vi "Initialize.vi"(7 "Option String":string="Simulate=1,RangeCheck=1,QueryInstrStatus=1,Cache=0", 8 "error in (no error)":errorcluster, 9 "btnReset":bool caption="Reset (F)", 10 "btnIdQuery":bool caption="Id Query (F)", 11 "ChromaAcLoad in":refnum<class "ChromaAcLoad.lvclass">) -> (0 "error out":errorcluster, 3 "ChromaAcLoad out":refnum<class "ChromaAcLoad.lvclass">)   [LabVIEW 2018, in "AcPwrPlugins.lvlib" / "ChromaAcLoad.lvclass"]
doc: "This VI estabilishes communication ot the instrument and optionally sets the initial state of the following session attributes:\n\n C63800_ATTR_RANGE_CHECK \n C63800_ATTR_QUERY_INSTR_STATUS \n C63800_ATTR_CACHE \n C63800_ATTR_SIMULATE \n C63800_ATTR_RECORD_COERCIONS \n\n- Opens a session to the specified device using the interface and address you specify for the Resource Name parameter.\n\n- If the ID Query parameter is set to VI_TRUE, this function queries the instrument ID and checks that it is valid for this instrument driver.\n\n- If the Reset parameter is set to VI_TRUE, this function resets the instrument to a known state.\n\n- Sends initialization commands to set the instrument to the state necessary for the operation of the instrument driver.\n\n- Returns a ViSession handle that you use to identify the instrument in all subsequent instrument driver function calls.\n\nNote: This function creates a new session each time you invoke it. Although you can open more than one IVI session for the same resource, it is best not to do so. You can use the same session in multiple program threads. You can use the C63800_LockSession and C63800_UnlockSession functions to protect sections of code that require exclusive access to the resource."
uses:
  ChromaAcLoad.lvclass
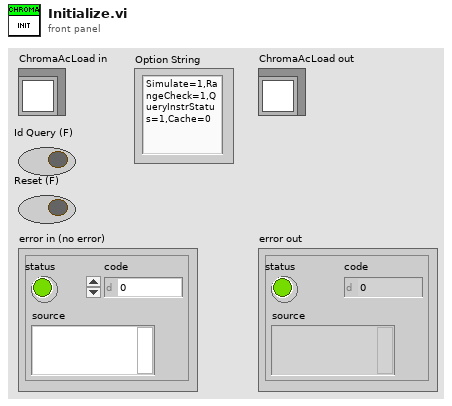
[diagram p1: front panel]
types:
  T1 = cluster{"f":bool, "Instrument Handle out":refnum<k15>}[]
  T2 = typedef "AcPwrPlugins.lvlib/ChromaAcLoad.lvclass/DeviceProperties.ctl" = cluster{"Frequency (Hz)":dbl, "Phases":cluster{"Handle":string, "Name":string, "Phase Select":i32, "option string ":string, "id query (Yes)":bool, "reset device (Yes)":bool, "LC":cluster{"C (uF)":i32, "L (uH)":i32, "RS (Ohm)":dbl, "RL (Ohm)":dbl}, "Load Current (A/Arms)":dbl, "Load Voltage (V/Vrms)":dbl, "Load Power (W)":dbl, "Load Resistance (Ohms)":dbl, "Load Current Peak (A)":dbl, "Load Current Limit (A/Arms)":dbl, "Slew Rate":cluster{"Rise Slew Rate (Units/S)":i32, "Fall Slew Rate (Units/S)":i32}, "Load Short Circuited":bool, "Line Synchronization":bool, "Priority":enum16{"CF Only", "PF Only", "Both (CF)", "Both (PF)"}, "Crest Factor":dbl, "Power Factor":dbl, "Connected":bool, "Voltage Range (V)":dbl[], "Timing":cluster{"TimingOn":enum16{""}, "Hours":u32, "Minutes":u32, "Seconds":dbl, "CutoffVoltage":dbl}}[], "Configuration Mode":enum16{"Constant Voltage (DC)", "Constant Power (DC)", "Constant Power (AC)", "Constant Current (DC)", "Constant Current (AC)", "Constant Resistance (DC)", "Constant Resistance (AC)", "Rectified Mode (DC)", "Inrush (AC)", "RLC CP (AC)", "RLC (AC)"}}[]
  T3 = cluster{"Handle":string, "Name":string, "Phase Select":i32, "option string ":string, "id query (Yes)":bool, "reset device (Yes)":bool, "LC":cluster{"C (uF)":i32, "L (uH)":i32, "RS (Ohm)":dbl, "RL (Ohm)":dbl}, "Load Current (A/Arms)":dbl, "Load Voltage (V/Vrms)":dbl, "Load Power (W)":dbl, "Load Resistance (Ohms)":dbl, "Load Current Peak (A)":dbl, "Load Current Limit (A/Arms)":dbl, "Slew Rate":cluster{"Rise Slew Rate (Units/S)":i32, "Fall Slew Rate (Units/S)":i32}, "Load Short Circuited":bool, "Line Synchronization":bool, "Priority":enum16{"CF Only", "PF Only", "Both (CF)", "Both (PF)"}, "Crest Factor":dbl, "Power Factor":dbl, "Connected":bool, "Voltage Range (V)":dbl[], "Timing":cluster{"TimingOn":enum16{""}, "Hours":u32, "Minutes":u32, "Seconds":dbl, "CutoffVoltage":dbl}}[]
  T4 = cluster{"f":bool, "Instrument Handle out":refnum<k15>}
  T5 = cluster{"Handle":string, "Name":string, "Phase Select":i32, "option string ":string, "id query (Yes)":bool, "reset device (Yes)":bool, "LC":cluster{"C (uF)":i32, "L (uH)":i32, "RS (Ohm)":dbl, "RL (Ohm)":dbl}, "Load Current (A/Arms)":dbl, "Load Voltage (V/Vrms)":dbl, "Load Power (W)":dbl, "Load Resistance (Ohms)":dbl, "Load Current Peak (A)":dbl, "Load Current Limit (A/Arms)":dbl, "Slew Rate":cluster{"Rise Slew Rate (Units/S)":i32, "Fall Slew Rate (Units/S)":i32}, "Load Short Circuited":bool, "Line Synchronization":bool, "Priority":enum16{"CF Only", "PF Only", "Both (CF)", "Both (PF)"}, "Crest Factor":dbl, "Power Factor":dbl, "Connected":bool, "Voltage Range (V)":dbl[], "Timing":cluster{"TimingOn":enum16{""}, "Hours":u32, "Minutes":u32, "Seconds":dbl, "CutoffVoltage":dbl}}
  T6 = cluster{"Frequency (Hz)":dbl, "Phases":cluster{"Handle":string, "Name":string, "Phase Select":i32, "option string ":string, "id query (Yes)":bool, "reset device (Yes)":bool, "LC":cluster{"C (uF)":i32, "L (uH)":i32, "RS (Ohm)":dbl, "RL (Ohm)":dbl}, "Load Current (A/Arms)":dbl, "Load Voltage (V/Vrms)":dbl, "Load Power (W)":dbl, "Load Resistance (Ohms)":dbl, "Load Current Peak (A)":dbl, "Load Current Limit (A/Arms)":dbl, "Slew Rate":cluster{"Rise Slew Rate (Units/S)":i32, "Fall Slew Rate (Units/S)":i32}, "Load Short Circuited":bool, "Line Synchronization":bool, "Priority":enum16{"CF Only", "PF Only", "Both (CF)", "Both (PF)"}, "Crest Factor":dbl, "Power Factor":dbl, "Connected":bool, "Voltage Range (V)":dbl[], "Timing":cluster{"TimingOn":enum16{""}, "Hours":u32, "Minutes":u32, "Seconds":dbl, "CutoffVoltage":dbl}}[], "Configuration Mode":enum16{"Constant Voltage (DC)", "Constant Power (DC)", "Constant Power (AC)", "Constant Current (DC)", "Constant Current (AC)", "Constant Resistance (DC)", "Constant Resistance (AC)", "Rectified Mode (DC)", "Inrush (AC)", "RLC CP (AC)", "RLC (AC)"}}
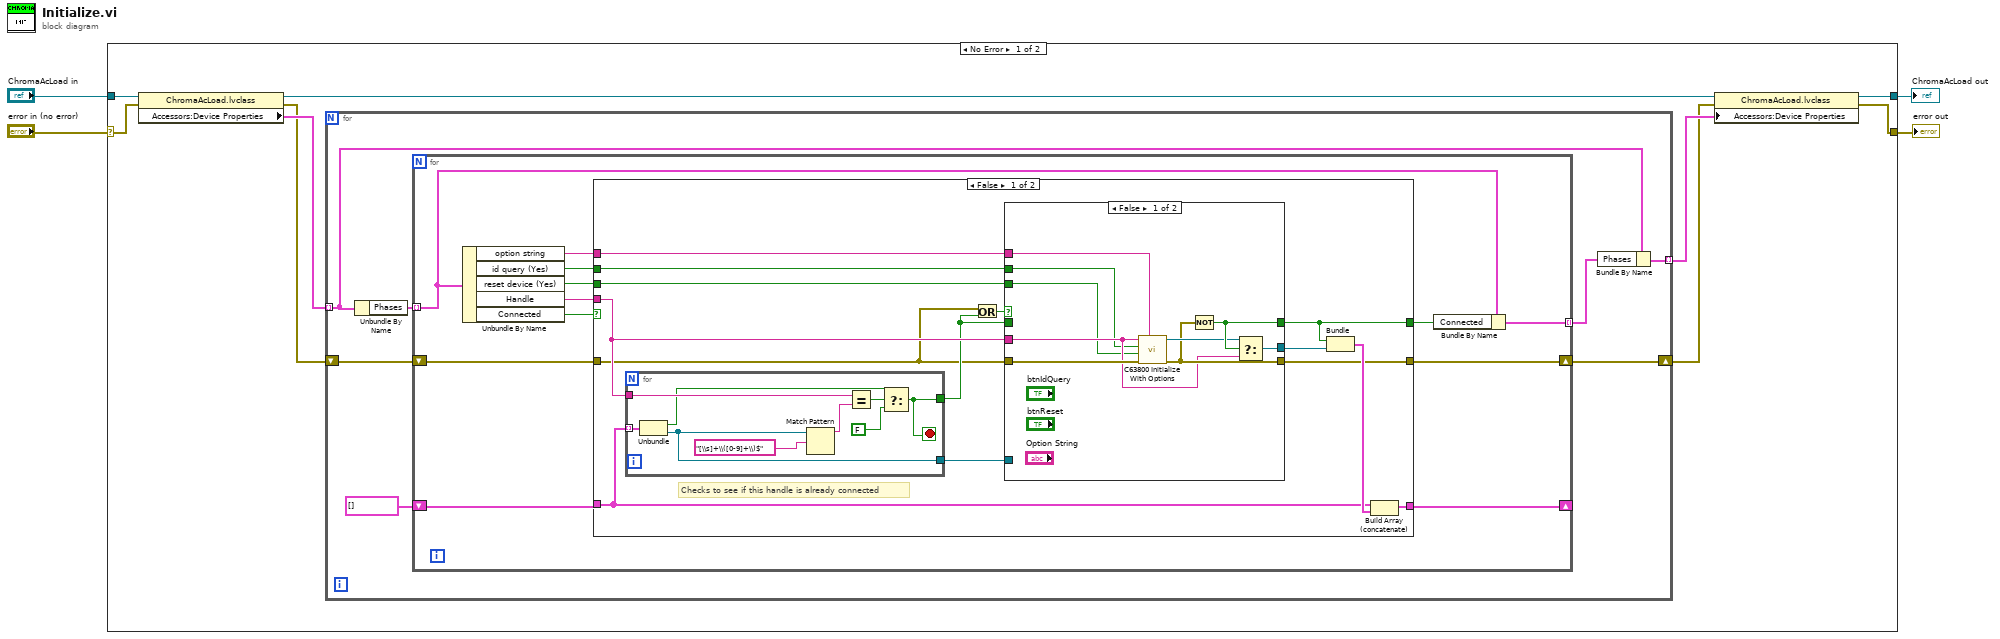
[diagram p0: block diagram]
diagram:
  n1 = case shown="No Error" "error in (no error)" {
    selector: "error in (no error)" -> [w12 w72]
    tunnel: "ChromaAcLoad in" -> [w13 w71]
    tunnel: [w10 w71] -> w2
    tunnel: [w5 w72] -> w1
    frame No Error {
      n2 = property class="ChromaAcLoad.lvclass"(reference=w13, error in=w12) -> (reference out=w11:refnum<class "ChromaAcLoad.lvclass">, error out=w7:errorcluster, "Accessors:Device Properties"=w9:T2)
      n3 = for {
        tunnel: w9 -> [w20] mode=indexing
        tunnel: [w19] -> w8 mode=indexing
        shift-right: [w14] -> w6
        shift-left: w7 -> [w18]
        n4 = Unbundle By Name(w20) -> ("Phases"=w17:T3)
        n5 = for {
          shift-right: [w31] -> w14
          shift-left: w18 -> [w32]
          tunnel: w17 -> [w25] mode=indexing
          shift-right: [w29] -> _
          shift-left: T1 [] -> [w30]
          tunnel: [w24] -> w15 mode=indexing
          n6 = Unbundle By Name(w25) -> ("option string"=w23:string, "id query (Yes)"=w22:bool, "reset device (Yes)"=w21:bool, "Handle"=w28:string, "Connected"=w27:bool)
          n7 = case shown="False" w27 {
            selector: w27 -> [_ w70]
            tunnel: [w37 w70] -> w26
            tunnel: w28 -> [w46 _]
            tunnel: [w38 w69] -> w31
            tunnel: w32 -> [w36 w69]
            tunnel: w30 -> [w39 w68]
            tunnel: [w43 w68] -> w29
            tunnel: w23 -> [w35 _]
            tunnel: w22 -> [w34 _]
            tunnel: w21 -> [w33 _]
            frame False {
              # "Checks to see if this handle is already connected"
              n8 = for {
                tunnel: w46 -> [w55]
                tunnel: [w53] -> w44
                tunnel: w39 -> [w49] mode=indexing
                tunnel: [w47] -> w40
                stop <- w53 stop-if-true
                n9 = Unbundle(w49) -> ("f"=w48:bool, "Instrument Handle out"=w47:refnum<k15>)
                n10 = Match Pattern(string=w47, regular expression="[\\s]+\\([0-9]+\\)$") -> (before substring=w51:string)  [unwired: 1 in, 3 out]
                n11 = Equal?(x=w55, y=w51) -> (x = y?=w54:bool)
                n12 = Select(t=w48, s=w54, f=FALSE) -> (s? t:f=w53:bool)
              }
              n13 = Or(x=w36, y=w44) -> (x .or. y?=w45:bool)
              n14 = case shown="False" w45 {
                tunnel: [w63 w66] -> w37
                tunnel: w46 -> [w59 _]
                tunnel: w36 -> [w60 w67]
                tunnel: [w61 w67] -> w38
                tunnel: w44 -> [_ w66]
                tunnel: [w64 w65] -> w42
                tunnel: w40 -> [_ w65]
                tunnel: w35 -> [w58 _]
                tunnel: w34 -> [w57 _]
                tunnel: w33 -> [w56 _]
                frame False {
                  n15 = call <instrlib>:"C63800 Initialize With Options.vi"("Option String"=w58, "error in (no error)"=w60, "Reset Device"=w56, "ID Query"=w57, "Resource Name"=w59) -> ("error out"=w61:errorcluster, "Instrument Handle out"=w62:refnum<k15>)  [unwired: 5 in]
                  n16 = Not(x=w61) -> (.not. x?=w63:bool)
                  n17 = Select(t=w62, s=w63, f=w59) -> (s? t:f=w64:refnum<k15>)
                }
                frame True {
                }
              }
              n18 = Bundle("f"=w37, "Instrument Handle out"=w42) -> (w41:T4)  [unwired: 1 in]
              n19 = Build Array (concatenate)(w39, w41) -> (w43:T1)
            }
            frame True {
            }
          }
          n20 = Bundle By Name(cluster=w25, "Connected"=w26) -> (w24:T5)
        }
        n21 = Bundle By Name(cluster=w20, "Phases"=w15) -> (w19:T6)
      }
      n22 = property class="ChromaAcLoad.lvclass"(reference=w11, error in=w6, "Accessors:Device Properties"=w8) -> (reference out=w10:refnum<class "ChromaAcLoad.lvclass">, error out=w5:errorcluster)
    }
    frame Error {
    }
  }
  "error out" <- w1
  "ChromaAcLoad out" <- w2
